vi "NTJ_Convert String to NT Numeric Array Buffer.vi"(11 "LV Buffer":string) -> (3 "NT Buffer":string)   [LabVIEW 2019]
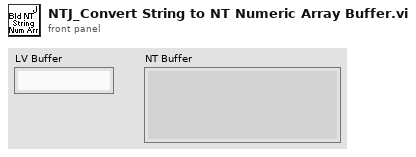
[diagram p1: front panel]
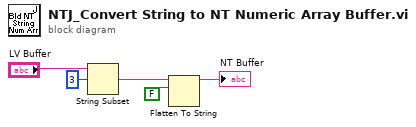
[diagram p0: block diagram]
diagram:
  n1 = String Subset(string="LV Buffer", offset (0)=3) -> (substring=w3:string)  [unwired: 1 in]
  n2 = Flatten To String(anything=w3, prepend array or string size? (T)=FALSE) -> (data string=→"NT Buffer":string)  [unwired: 2 in, 2 out]
